vi "Set Source Count.vi"(7 "Source Count":i32=1, 8 "error in (no error)":errorcluster, 11 "BuildSpec in":refnum<vi>) -> (0 "error out":errorcluster, 3 "BuildSpec out":refnum<vi>)   [LabVIEW 2019, in "Project Sync Tools.lvclass"]
uses:
  Project Sync Tools.lvclass
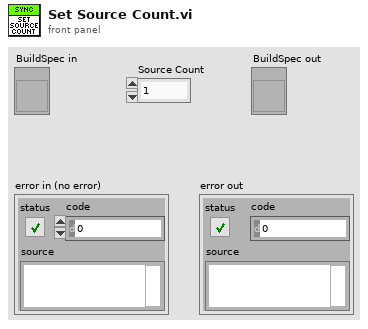
[diagram p1: front panel]
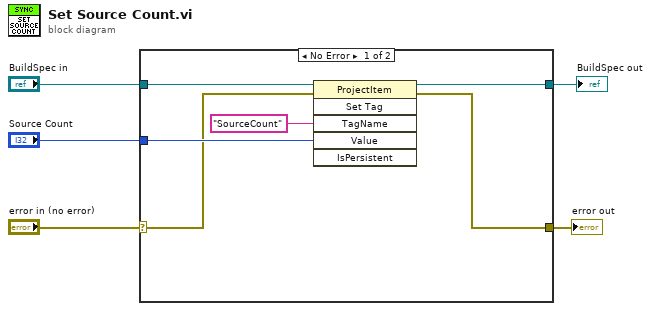
[diagram p0: block diagram]
diagram:
  n1 = case shown="No Error" "error in (no error)" {
    selector: "error in (no error)" -> [w6 w12]
    tunnel: "BuildSpec in" -> [w11 w13]
    tunnel: [w10 w12] -> w4
    tunnel: "Source Count" -> [w9 _]
    tunnel: [w7 w13] -> w2
    frame No Error {
      n2 = invoke class="ProjectItem" method="Set Tag"(reference=w11, error in=w6, "TagName"="SourceCount", "Value"=w9) -> (reference out=w7:refnum<vi>, error out=w10:errorcluster)  [unwired: 2 in, 4 out]
    }
    frame Error {
    }
  }
  "error out" <- w4
  "BuildSpec out" <- w2
